vi "process.vi"(8 "error in (no error)":errorcluster, 11 "Dependencies in":refnum<class "Dependencies.lvclass">) -> (0 "error out":errorcluster, 3 "Dependencies out":refnum<class "Dependencies.lvclass">)   [LabVIEW 2016, in "Dependencies.lvclass"]
uses:
  Dependencies.lvclass
  C:/LSST_TS/SystemSW/ct_tools/ProjectItem/ProjectItem.lvclass
  ProjectItem/ProjectItem.lvclass/ProjectItem.ctl
  Search/Search.lvclass/Search.ctl
  IProjectItemFactory/IProjectItemFactory.lvclass
  ProjectItem/ProjectItem.lvclass
  Project/Project.lvclass
  Search/Search.lvclass
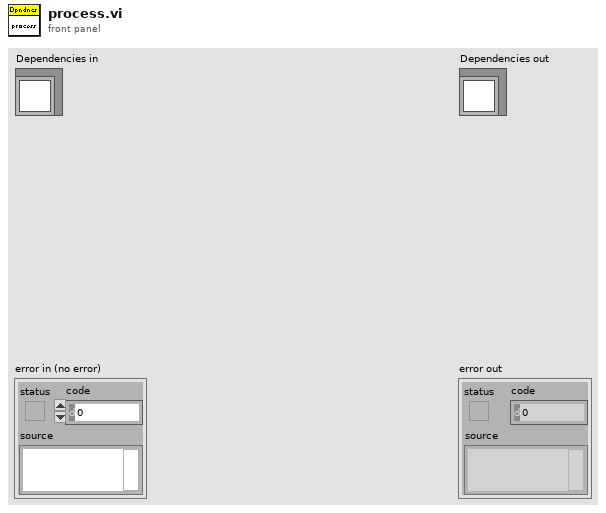
[diagram p1: front panel]
types:
  T1 = cluster{"OldLibrary":string, "NewLibrary":string}
  T2 = typedef "ProjectItemSelection.ctl" = enum16{"Default", "Dependencies", "Folder", "Library", "LVClass", "VI"}
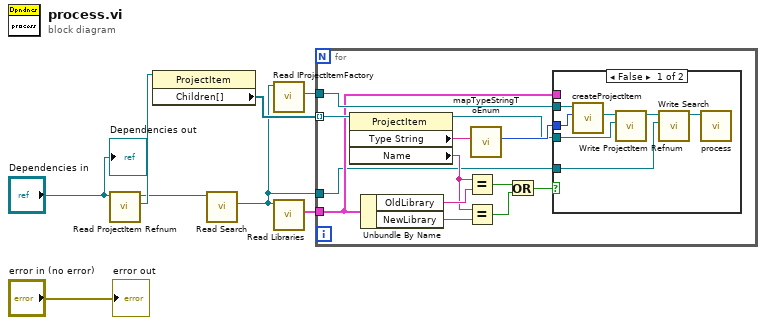
[diagram p0: block diagram]
diagram:
  n1 = call "Read ProjectItem Refnum.vi"("ProjectItem in"="Dependencies in") -> ("ProjectItem Refnum"=w6:refnum<vi>, "ProjectItem out"=w4:refnum<class "Dependencies.lvclass">)  [unwired: 9 in]
  n2 = property class="ProjectItem"(reference=w6) -> ("Children[]"=w5:refnum<vi>[])  [unwired: 1 in, 2 out]
  n3 = call "Read Search.vi"("ProjectItem in"=w4) -> ("Search"=w1:refnum<class "Search.lvclass">)  [unwired: 9 in, 1 out]
  n4 = call "Read IProjectItemFactory.vi"("ProjectItem in"=w1) -> ("IProjectItemFactory"=w2:refnum<class "IProjectItemFactory.lvclass">)  [unwired: 9 in, 1 out]
  n5 = call "Read Libraries.vi"("ProjectItem in"=w1) -> ("Libraries"=w3:T1)  [unwired: 9 in, 1 out]
  n6 = for {
    tunnel: w5 -> [w21] mode=indexing
    tunnel: w2 -> [w17]
    tunnel: w3 -> [w16]
    tunnel: w1 -> [w9]
    n7 = property class="ProjectItem"(reference=w21) -> (reference out=w18:refnum<vi>, "Type String"=w20:string, "Name"=w13:string)  [unwired: 1 in, 1 out]
    n8 = Unbundle By Name(w16) -> ("OldLibrary"=w15:string, "NewLibrary"=w14:string)
    n9 = Equal?(x=w13, y=w15) -> (x = y?=w12:bool)
    n10 = Equal?(x=w13, y=w14) -> (x = y?=w11:bool)
    n11 = call "mapTypeStringToEnum.vi"("Type String"=w20) -> ("ProjectItemSelection"=w19:T2)  [unwired: 8 in, 2 out]
    n12 = Or(x=w12, y=w11) -> (x .or. y?=w10:bool)
    n13 = case shown="False" w10 {
      tunnel: w19 -> [w28 _]
      tunnel: w18 -> [w26 _]
      tunnel: w17 -> [w25 _]
      tunnel: w16 -> [_ _]
      tunnel: w9 -> [w24 _]
      frame False {
        n14 = call-dynamic "createProjectItem.vi"("ProjectItemSelection"=w28, "IProjectItemFactory in"=w25) -> ("ProjectItem"=w27:refnum<class "ProjectItem.lvclass">)  [unwired: 7 in, 2 out]
        n15 = call "Write ProjectItem Refnum.vi"("ProjectItem Refnum"=w26, "ProjectItem in"=w27) -> ("ProjectItem out"=w23:refnum<class "ProjectItem.lvclass">)  [unwired: 9 in]
        n16 = call "Write Search.vi"("Search"=w24, "ProjectItem in"=w23) -> ("ProjectItem out"=w22:refnum<class "ProjectItem.lvclass">)  [unwired: 9 in]
        n17 = call-dynamic "process.vi"("ProjectItem in"=w22) -> ()  [unwired: 9 in, 2 out]
      }
      frame True {
      }
    }
  }
  "error out" <- "error in (no error)"
  "Dependencies out" <- "Dependencies in"
